vi "Controls to Commands.vi"(9 "Input Cluster 2":T3) -> (3 "Output Cluster 2":T1)   [LabVIEW 2015]
uses:
  Joytsick/Joytstick Controls Type.ctl
  Joytsick/Controls to Cmmnds Output Clust.ctl
  Joytsick/Controls to Cmmnds Type.ctl
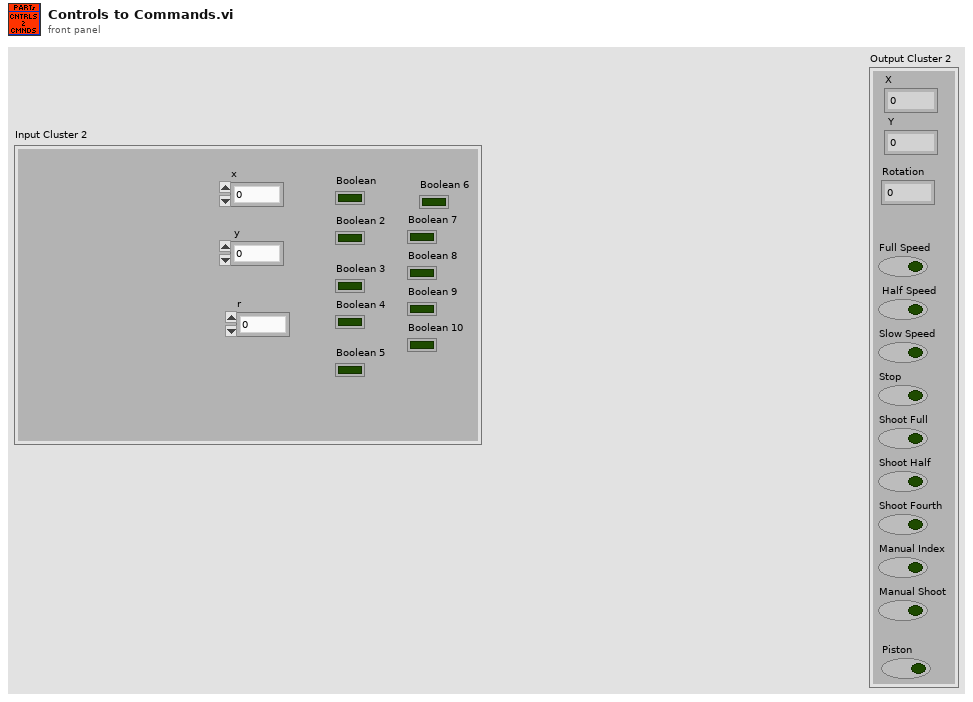
[diagram p1: front panel]
types:
  T1 = typedef "Controls to Cmmnds Output Clust.ctl" = cluster{"X ":dbl, " Y":dbl, "Rotation":dbl, "Full Speed":bool, " Half Speed":bool, "Slow Speed":bool, "Stop":bool, "Shoot Full":bool, "Shoot Half":bool, "Shoot Fourth":bool, "Manual Index":bool, "Manual Shoot":T2, "Piston":T2}
  T2 = typedef "Controls to Cmmnds Type.ctl" = bool
  T3 = typedef "Joytstick Controls Type.ctl" = cluster{"x":dbl, " y":dbl, "r":dbl, "Boolean":bool, "Boolean 2":bool, "Boolean 3":bool, "Boolean 4":bool, "Boolean 5":bool, "Boolean 6":bool, "Boolean 7":bool, "Boolean 8":bool, "Boolean 9":bool, "Boolean 10":bool}
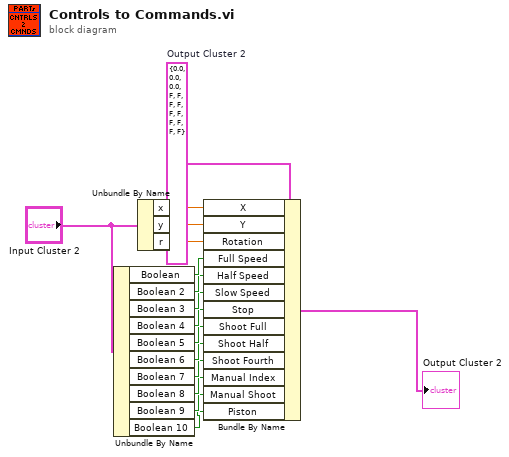
[diagram p0: block diagram]
diagram:
  w3 = T1 {"X "=0.0, " Y"=0.0, "Rotation"=0.0, "Full Speed"=FALSE, " Half Speed"=FALSE, "Slow Speed"=FALSE, "Stop"=FALSE, "Shoot Full"=FALSE, "Shoot Half"=FALSE, "Shoot Fourth"=FALSE, "Manual Index"=FALSE, "Manual Shoot"=FALSE, "Piston"=FALSE}  # Output Cluster 2
  n1 = Unbundle By Name("Input Cluster 2") -> ("Boolean"=w12:bool, "Boolean 2"=w11:bool, "Boolean 3"=w10:bool, "Boolean 4"=w9:bool, "Boolean 5"=w8:bool, "Boolean 6"=w7:bool, "Boolean 7"=w6:bool, "Boolean 8"=w5:bool, "Boolean 9"=w4:bool, "Boolean 10"=w1:bool)
  n2 = Unbundle By Name("Input Cluster 2") -> ("x"=w15:dbl, "y"=w14:dbl, "r"=w13:dbl)
  n3 = Bundle By Name(cluster=w3, "X"=w15, "Y"=w14, "Rotation"=w13, "Full Speed"=w12, "Half Speed"=w11, "Slow Speed"=w10, "Stop"=w9, "Shoot Full"=w8, "Shoot Half"=w7, "Shoot Fourth"=w6, "Manual Index"=w5, "Manual Shoot"=w4, "Piston"=w1) -> (→"Output Cluster 2":T1)
